vi "ini_save_double_multi.vi"(7 "section":string, 8 "error in":errorcluster, 9 "doubles":dbl[](array[numeric]), 10 "keys (multiline string)":string, 11 "refnum in":T1) -> (0 "error out":errorcluster, 2 "found?":bool[](array[boolean]), 3 "refnum out":T1)   [LabVIEW 2013]
uses:
  <vilib>/Utility/config.llb/Config Data RefNum.ctl
  <vilib>/Utility/config.llb/Write Key (Double).vi
  <vilib>/Utility/config.llb/NI_LVConfig.lvlib
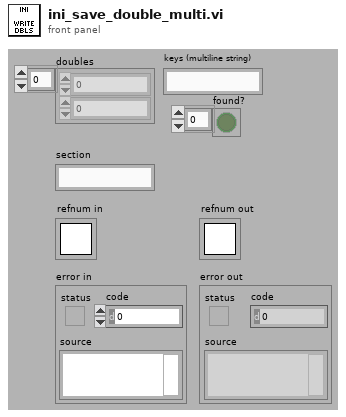
[diagram p1: front panel]
types:
  T1 = typedef "NI_LVConfig.lvlib/Config Data RefNum.ctl" = refnum<k1>
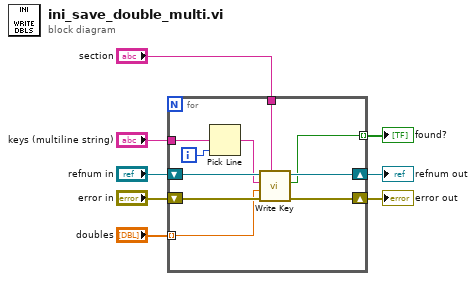
[diagram p0: block diagram]
diagram:
  n1 = for {
    tunnel: "section" -> [w14]
    tunnel: "keys (multiline string)" -> [w13]
    shift-right: [w15] -> w5
    shift-left: "refnum in" -> [w16]
    shift-right: [w17] -> w7
    shift-left: "error in" -> [w18]
    tunnel: "doubles" -> [w10] mode=indexing
    tunnel: [w9] -> w1 mode=indexing
    i -> [w11]
    n2 = Pick Line(multi-line string=w13, line index=w11) -> (output string=w12:string)  [unwired: 1 in]
    n3 = call-poly <vilib>:"Write Key.vi"("section"=w14, "error in (no error)"=w18, "value"=w10, "key"=w12, "refnum"=w16) -> ("error out"=w17:errorcluster, "found?"=w9:bool, "refnum out"=w15:T1)  [unwired: 4 in]
  }
  "error out" <- w7
  "refnum out" <- w5
  "found?" <- w1
